vi "例6-7.vi"() -> ()   [LabVIEW 2019]
uses:
  <vilib>/Analysis/1siggen.llb/Ramp Pattern by Samples.vi
  <vilib>/Analysis/2dsp.llb/1D Convolution (DBL).vi
  <vilib>/Analysis/NI_AALBase.lvlib
  <vilib>/Analysis/NI_AALPro.lvlib
panel:
  out "波形图2":dbl[](graph)
  out "波形图1":dbl[](graph)
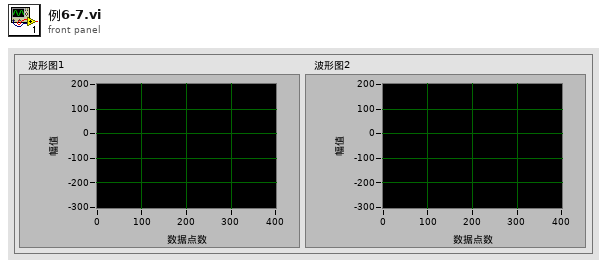
[diagram p1: front panel]
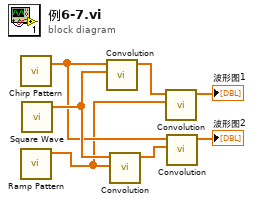
[diagram p0: block diagram]
diagram:
  n1 = call <vilib>:"Chirp Pattern.vi"() -> ("Chirp Pattern"=w5:dbl[])  [unwired: 4 in, 1 out]
  n2 = call-poly <vilib>:"Ramp Pattern.vi"() -> ("Ramp Pattern"=w1:dbl[])  [unwired: 10 in, 1 out]
  n3 = call <vilib>:"Square Wave.vi"() -> ("square wave"=w6:dbl[])  [unwired: 6 in, 2 out]
  n4 = call-poly <vilib>:"Convolution.vi"("Y"=w6, "X"=w5) -> ("X * Y"=w7:dbl[])  [unwired: 8 in, 1 out]
  n5 = call-poly <vilib>:"Convolution.vi"("Y"=w1, "X"=w6) -> ("X * Y"=w4:dbl[])  [unwired: 8 in, 1 out]
  n6 = call-poly <vilib>:"Convolution.vi"("Y"=w1, "X"=w7) -> ("X * Y"=→"波形图1":dbl[])  [unwired: 8 in, 1 out]
  n7 = call-poly <vilib>:"Convolution.vi"("Y"=w4, "X"=w5) -> ("X * Y"=→"波形图2":dbl[])  [unwired: 8 in, 1 out]
